vi "Compile FIU.vi"(8 "error in (no error)":errorcluster, 10 "SLSC Compiled in":T1, 11 "Device Item Ref in":T2 format="%.0x") -> (0 "error out":errorcluster, 2 "SLSC Compiled out":T1, 3 "Device Item Ref out":T2 format="%.0x")   [LabVIEW 2013, in "SLSC configuration System Explorer.lvlib"]
uses:
  SLSC configuration System Explorer.lvlib
  <vilib>/NI Veristand/Custom Device API/Custom Device Item Ref.ctl
  Shared/SLSC compiled.ctl
  Shared/Card Postion.ctl
  Shared/FIU compiled.ctl
  <vilib>/NI Veristand/Custom Device API/Data Access Type.ctl
  Shared/Constants.vi
  <vilib>/NI Veristand/Custom Device API/Get Item Property (Variant).vi
  <vilib>/NI Veristand/Custom Device API/Get Item Property (U16).vi
  <vilib>/NI Veristand/Custom Device Tools/Custom Device Utility Library/Custom Device Utility Library.lvlib
  Shared/SLSC configuration Shared.lvlib
  <vilib>/NI Veristand/Custom Device API/Custom Device API.lvlib
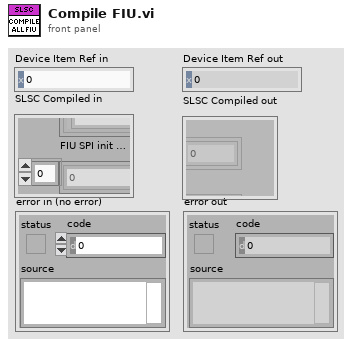
[diagram p1: front panel]
types:
  T1 = typedef "SLSC configuration Shared.lvlib/SLSC compiled.ctl" = cluster{"DIO SPI init FIFO elements":u32[], "FIU SPI read data ":cluster{"Previous channel values":dbl[], "Channel Indices":i32[], "FIFO bytes3_2":u32}[], "FIU SPI init FIFO elements":u32[]}
  T2 = typedef "Custom Device API.lvlib/Custom Device Item Ref.ctl" = u64
  T3 = typedef "SLSC configuration Shared.lvlib/FIU compiled.ctl" = cluster{"Channel old values":dbl[], "Channel data refs":i32[], "FIFO bytes3_2":u32}
  T4 = typedef "SLSC configuration Shared.lvlib/Card Postion.ctl" = cluster{"Chassis #":u8, "Slot #":u8}
  T5 = typedef "Custom Device API.lvlib/Data Access Type.ctl" = enum16{"Read", "Write"}
  T6 = typedef "Custom Device API.lvlib/Custom Device Channel.ctl" = cluster{"Type":T7, "Units":string, "Default Value":dbl, "Faultable":bool, "Scalable":bool}
  T7 = typedef "Custom Device API.lvlib/Custom Device Channel Type.ctl" = enum16{"Input", "Output"}
  T8 = typedef "Custom Device API.lvlib/Data Reference.ctl" = i32
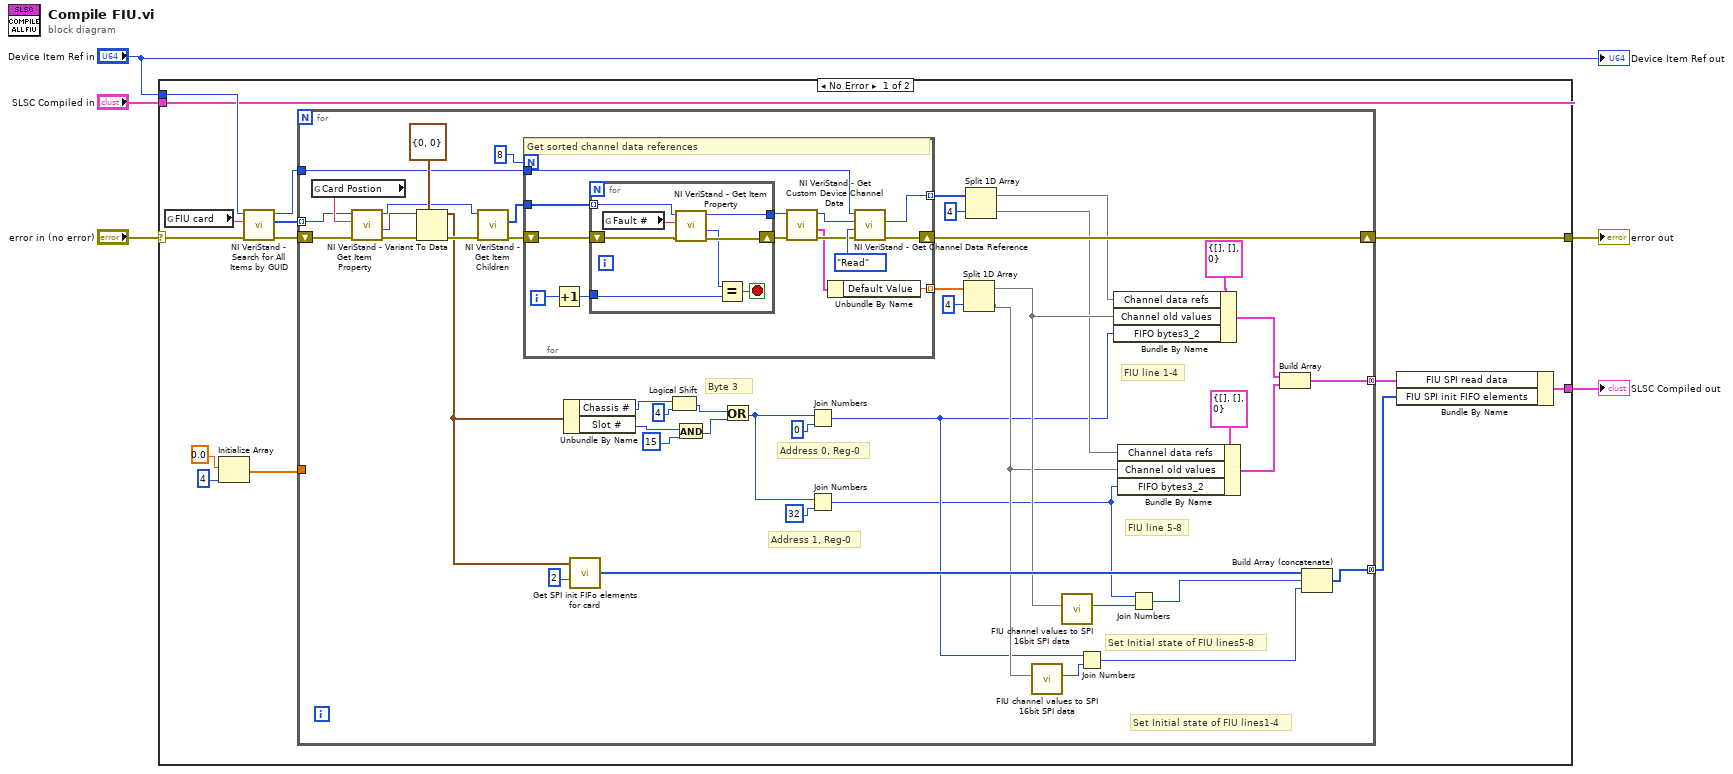
[diagram p0: block diagram]
diagram:
  n1 = case shown="No Error" "error in (no error)" {
    selector: "error in (no error)" -> [w7 w88]
    tunnel: [w15 w88] -> w5
    tunnel: "Device Item Ref in" -> [w14 _]
    tunnel: [w8 w87] -> w3
    tunnel: "SLSC Compiled in" -> [w6 w87]
    frame No Error {
      n2 = global read "Constants.vi" "FIU card"() -> (w19:string)
      n3 = Initialize Array(0.0 ("element"), 4 ("dimension size")) -> (w11:dbl[])
      n4 = call <vilib>:"NI VeriStand - Search for All Items by GUID.vi"("error in"=w7, "Item GUID"=w19, "Section Ref in"=w14) -> ("error out"=w18:errorcluster, "Item Refs"=w16:T2[], "Section Ref out"=w17:T2)  [unwired: 5 in, 1 out]
      n5 = for {
        tunnel: w17 -> [w48]
        tunnel: w16 -> [w50] mode=indexing
        tunnel: [w22] -> w9 mode=concatenating
        tunnel: w11 -> [_]
        shift-right: [w32] -> w15
        shift-left: w18 -> [w58]
        tunnel: [w39] -> w10 mode=concatenating
        # "Set Initial state of FIU lines5-8"
        # "Set Initial state of FIU lines1-4"
        # "Address 1, Reg-0"
        # "Address 0, Reg-0"
        # "FIU line 5-8"
        # "FIU line 1-4"
        # "Byte 3"
        n6 = global read "Constants.vi" "Card Postion"() -> (w57:string)
        n7 = call-poly <vilib>:"NI VeriStand - Get Item Property.vi"("error in (no error)"=w58, "Property Name"=w57, "Item Ref in"=w50) -> ("error out"=w60:errorcluster, "Value"=w61:variant, "Item Ref out"=w49:T2)  [unwired: 5 in, 1 out]
        n8 = Variant To Data(error in=w60, type=T4 {"Chassis #"=0, "Slot #"=0} ("Card Position"), Variant=w61) -> (data=w47:T4, error out=w59:errorcluster)
        n9 = call <vilib>:"NI VeriStand - Get Item Children.vi"("error in (no error)"=w59, "Item Ref in"=w49) -> ("error out"=w33:errorcluster, "Child Refs"=w63:T2[])  [unwired: 6 in, 2 out]
        n10 = for {
          N: 8 -> [_]
          tunnel: w63 -> [w77]
          tunnel: w48 -> [w75]
          tunnel: [w68] -> w38 mode=indexing
          tunnel: [w67] -> w35 mode=indexing
          shift-right: [w66] -> w32
          shift-left: w33 -> [w65]
          i -> [w78]
          # "Get sorted channel data references"
          n11 = Increment(x=w78) -> (x+1=w73:i32)
          n12 = for {
            shift-right: [w85] -> w76
            shift-left: w65 -> [w86]
            tunnel: w73 -> [w81]
            tunnel: w77 -> [w83] mode=indexing
            tunnel: [w79] -> w71
            stop <- w80 stop-if-true
            n13 = global read "Constants.vi" "Fault #"() -> (w84:string)
            n14 = call-poly <vilib>:"NI VeriStand - Get Item Property.vi"("error in (no error)"=w86, "Property Name"=w84, "Item Ref in"=w83) -> ("error out"=w85:errorcluster, "Value"=w82:u16, "Item Ref out"=w79:T2)  [unwired: 5 in, 1 out]
            n15 = Equal?(x=w82, y=w81) -> (x = y?=w80:bool)
          }
          n16 = call <vilib>:"NI VeriStand - Get Custom Device Channel Data.vi"("error in (no error)"=w76, "Channel Ref in"=w71) -> ("error out"=w72:errorcluster, "Channel"=w69:T6, "Channel Ref out"=w70:T2)  [unwired: 4 in, 3 out]
          n17 = Unbundle By Name(w69) -> ("Default Value"=w67:dbl)
          n18 = call <vilib>:"NI VeriStand - Get Channel Data Reference.vi"("error in (no error)"=w72, "Access"=Data_Access_Type."Read", "Channel Ref in"=w70, "Device Ref in"=w75) -> ("error out"=w66:errorcluster, "Channel Data Reference"=w68:T8)  [unwired: 5 in, 1 out]
        }
        n19 = Unbundle By Name(w47) -> ("Chassis #"=w56:u8, "Slot #"=w54:u8)
        n20 = call "Get SPI init FIFo elements for card.vi"("Num of SPI ICs"=u8 2, "Card Position"=w47) -> ("init FIFO elements"=w31:u32[])  [unwired: 9 in]
        n21 = Logical Shift(y=w56, x=u8 4) -> (x << y=w52:u8)
        n22 = And(x=w54, y=u8 15) -> (x .and. y?=w51:u8)
        n23 = Or(x=w52, y=w51) -> (x .or. y?=w42:u8)
        n24 = Join Numbers(hi=u8 0 ("lo"), lo=w42) -> ((hi.lo)=w25:u16)
        n25 = Join Numbers(hi=w42, lo=u8 32) -> ((hi.lo)=w24:u16)
        n26 = Split 1D Array(array=w35, index=4) -> (first subarray=w30:dbl[], second subarray=w27:dbl[])
        n27 = Split 1D Array(array=w38, index=4) -> (first subarray=w29:T8[], second subarray=w28:T8[])
        n28 = call "FIU channel values to SPI 16bit SPI data.vi"("FIU Channel values"=w27) -> ("data word"=w26:u16)  [unwired: 10 in]
        n29 = call "FIU channel values to SPI 16bit SPI data.vi"("FIU Channel values"=w30) -> ("data word"=w23:u16)  [unwired: 10 in]
        n30 = Join Numbers(hi=w25, lo=w26) -> ((hi.lo)=w20:u32)
        n31 = Bundle By Name(cluster=T3 {"Channel old values"=[], "Channel data refs"=[], "FIFO bytes3_2"=0} ("FIU SPI command"), "Channel data refs"=w29, "Channel old values"=w30, "FIFO bytes3_2"=w25) -> (w40:T3)
        n32 = Bundle By Name(cluster=T3 {"Channel old values"=[], "Channel data refs"=[], "FIFO bytes3_2"=0} ("FIU SPI command"), "Channel data refs"=w28, "Channel old values"=w27, "FIFO bytes3_2"=w24) -> (w34:T3)
        n33 = Join Numbers(hi=w24, lo=w23) -> ((hi.lo)=w21:u32)
        n34 = Build Array(w40, w34) -> (w39:T3[])
        n35 = Build Array (concatenate)(w31, w21, w20) -> (w22:u32[])
      }
      n36 = Bundle By Name(cluster=w6, "FIU SPI read data"=w10, "FIU SPI init FIFO elements"=w9) -> (w8:T1)
    }
    frame Error {
    }
  }
  "error out" <- w5
  "SLSC Compiled out" <- w3
  "Device Item Ref out" <- "Device Item Ref in"
